vi "PollMessages.vi"(8 "error in (no error)":errorcluster, 11 "PolledDriver in":refnum<class "PolledDriver.lvclass">) -> (0 "error out":errorcluster, 1 "disconnected":refnum<class "BaseMessage.lvclass">, 2 "connected":refnum<class "BaseMessage.lvclass">[](array[class]), 3 "PolledDriver out":refnum<class "PolledDriver.lvclass">)   [LabVIEW 2013, in "PolledDriver.lvclass"]
doc: "Returns an array of messages to send when polling the driver. Override with messages in derived drivers"
uses:
  PolledDriver.lvclass
  Message/BaseMessage/BaseMessage.lvclass
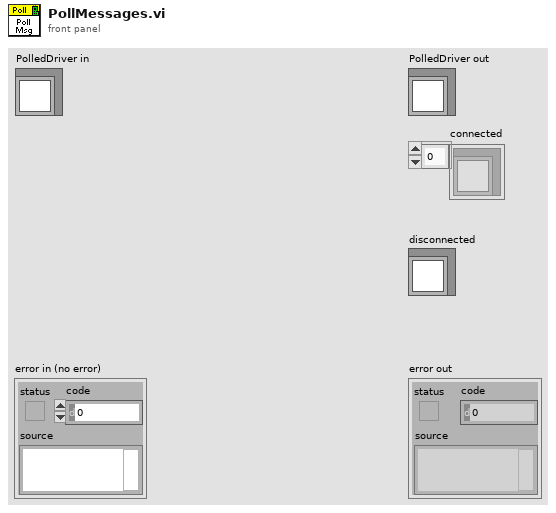
[diagram p1: front panel]
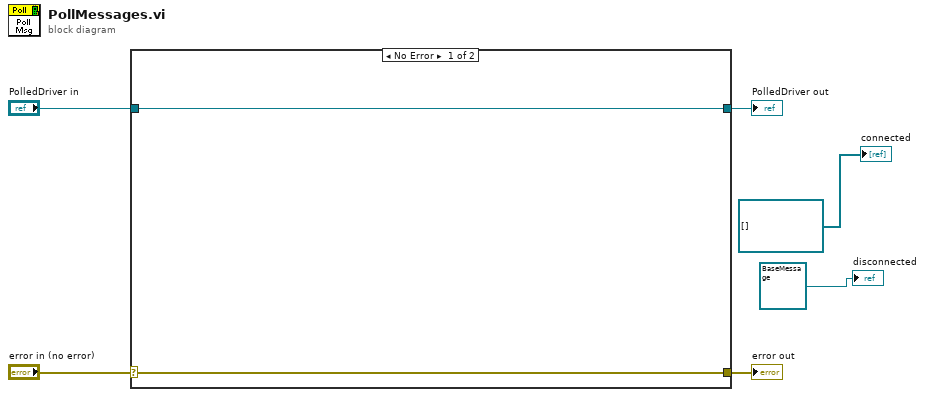
[diagram p0: block diagram]
diagram:
  n1 = case shown="No Error" "error in (no error)" {
    selector: "error in (no error)" -> [w7 w10]
    tunnel: [w7 w10] -> w5
    tunnel: [w8 w9] -> w3
    tunnel: "PolledDriver in" -> [w8 w9]
    frame No Error {
    }
    frame Error {
    }
  }
  "error out" <- w5
  "PolledDriver out" <- w3
  "connected" <- refnum<class "BaseMessage.lvclass">[] [] ("disconnected")
  "disconnected" <- refnum<class "BaseMessage.lvclass"> refnum ("BaseMessage.lvclass")
